vi "AutoFollowRelativeTrajectoryNEW.vi"(8 "error in (no error)":errorcluster, 9 "TimeOut (s)":dbl, 10 "End Orientation":dbl, 11 "Trajectory":T1 {"States"."POSE"."ROTATION"."SIN" format="%13.4f"; "States"."POSE"."ROTATION"."COS" format="%13.4f"; "States"."POSE"."ROTATION"."VALUE" format="%13.4f"; "States"."POSE"."TRANSLATION"."Y" format="%14.3f"; "States"."POSE"."TRANSLATION"."X" format="%14.3f"; "TotalTImeSecs" format="%20.3f"}) -> (0 "error out":errorcluster)   [LabVIEW 2023]
doc: "Wrapper class for drive straight"
uses:
  <vilib>/Rock Robotics/WPI/ThirdParty/JAS_Junk/TrajLib/TypeDef/TRAJECTORY.ctl
  <vilib>/Rock Robotics/WPI/ThirdParty/JAS_Junk/TrajLib/TypeDef/TRAJ_STATE.ctl
  <vilib>/Rock Robotics/WPI/ThirdParty/JAS_Junk/TrajLib/TypeDef/POSE2D.ctl
  <vilib>/Rock Robotics/WPI/ThirdParty/JAS_Junk/TrajLib/TypeDef/TRANSLATION2D.ctl
  <vilib>/Rock Robotics/WPI/ThirdParty/JAS_Junk/TrajLib/TypeDef/ROTATION2D.ctl
  <vilib>/Rock Robotics/WPI/ThirdParty/JAS_Junk/TrajLib/ChassisSpeeds_New.vi
  <vilib>/Rock Robotics/WPI/ThirdParty/JAS_Junk/TrajLib/Conv_Feet_Meters.vi
  <vilib>/Rock Robotics/WPI/ThirdParty/JAS_Junk/TrajLib/Conv_Deg_Radians.vi
  <vilib>/Utility/semaphor.llb/Obtain Semaphore Reference.vi
  <vilib>/Rock Robotics/WPI/ThirdParty/JAS_Junk/TrajLib/Timer_Reset.vi
  Drive/DriveGlobal.vi
  <vilib>/Rock Robotics/WPI/ThirdParty/JAS_Junk/TrajLib/Trajectory_Library.lvlib
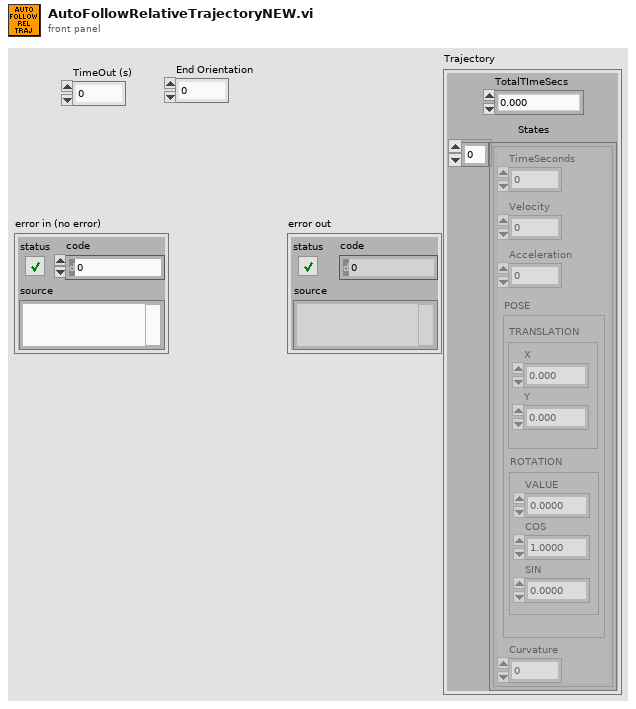
[diagram p1: front panel]
types:
  T1 = typedef "Trajectory_Library.lvlib/TRAJECTORY.ctl" = cluster{"TotalTImeSecs":dbl, "States":T2[]}
  T2 = typedef "Trajectory_Library.lvlib/TRAJ_STATE.ctl" = cluster{"TimeSeconds":dbl, "Velocity":dbl, "Acceleration":dbl, "POSE":T3, "Curvature":dbl}
  T3 = typedef "Trajectory_Library.lvlib/POSE2D.ctl" = cluster{"TRANSLATION":T4, "ROTATION":T5}
  T4 = typedef "Trajectory_Library.lvlib/TRANSLATION2D.ctl" = cluster{"X":dbl, "Y":dbl}
  T5 = typedef "Trajectory_Library.lvlib/ROTATION2D.ctl" = cluster{"VALUE":dbl, "COS":dbl, "SIN":dbl}
  T6 = typedef "Trajectory_Library.lvlib/TIMER.ctl" = cluster{"StartTime":dbl, "Accumulated TIme":dbl, "Running":bool, "semaphore":T7}
  T7 = typedef "Semaphore RefNum" = refnum<k1>
  T8 = typedef "Trajectory_Library.lvlib/CHASSIS_SPEEDS.ctl" = cluster{"vX":dbl, "vY":dbl, "vOmega":dbl}
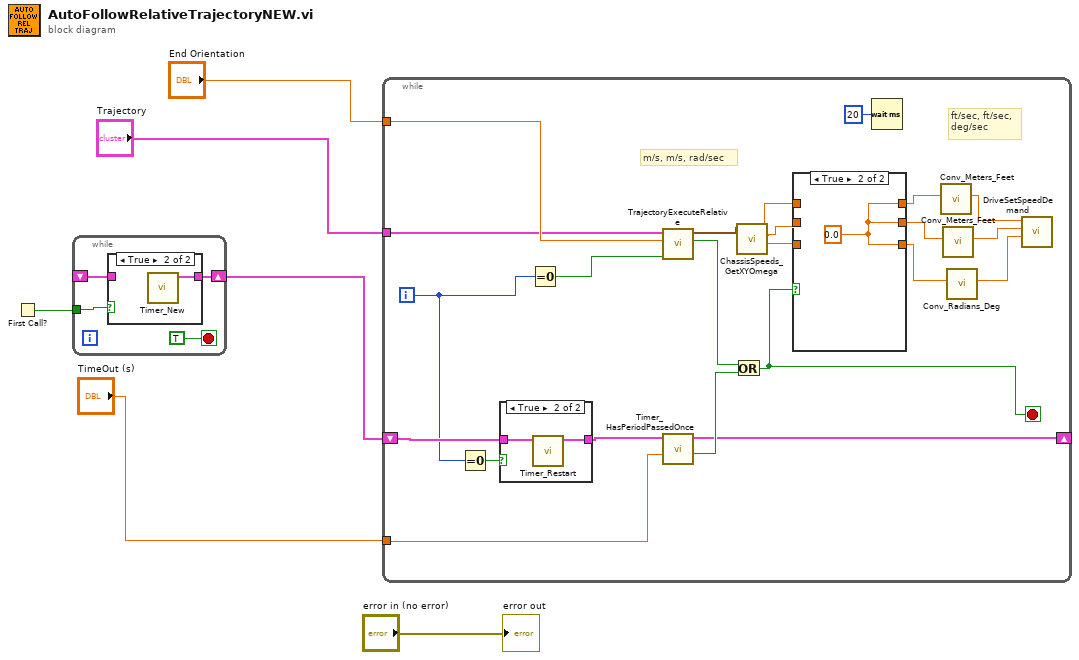
[diagram p0: block diagram]
diagram:
  n1 = First Call?() -> (First Call?: T/F=w2:bool)
  n2 = while {
    tunnel: w2 -> [w7]
    shift-right: [w10] -> w1
    shift-left: _ -> [w8]
    stop <- TRUE stop-if-true
    n3 = case shown="True" w7 {
      tunnel: [w11 w12] -> w10
      tunnel: w8 -> [w11 _]
      frame False {
      }
      frame True {
        n4 = call <vilib>:"Timer_New.vi"() -> ("TIMER"=w12:T6)  [unwired: 11 in]
      }
    }
  }
  n5 = while {
    tunnel: "TimeOut (s)" -> [w35]
    tunnel: "Trajectory" -> [w31]
    tunnel: "End Orientation" -> [w32]
    shift-right: [w15] -> _
    shift-left: w1 -> [w14]
    i -> [w13]
    stop <- w18 stop-if-true
    # "ft/sec, ft/sec,\ndeg/sec"
    # "m/s, m/s, rad/sec"
    n6 = Equal To 0?(x=w13) -> (x = 0?=w17:bool)
    n7 = case shown="True" w17 {
      tunnel: w14 -> [w36 w38]
      tunnel: [w36 w37] -> w16
      frame False {
      }
      frame True {
        n8 = call <vilib>:"Timer_Restart.vi"("in Timer"=w38) -> ("out Timer"=w37:T6)  [unwired: 10 in]
      }
    }
    n9 = Equal To 0?(x=w13) -> (x = 0?=w30:bool)
    n10 = call "TrajectoryExecuteRelative.vi"("Init"=w30, "End Relative\nOrientation Deg"=w32, "Trajectory"=w31) -> ("Done"=w29:bool, "Chassis Velocity Target Met,Met,Rad"=w25:T8)  [unwired: 6 in, 1 out]
    n11 = call <vilib>:"Timer_HasPeriodPassedOnce.vi"("Period"=w35, "in Timer"=w16) -> ("Expired"=w34:bool, "out Timer"=w15:T6)  [unwired: 7 in, 1 out]
    n12 = Or(x=w29, y=w34) -> (x .or. y?=w18:bool)
    n13 = call <vilib>:"ChassisSpeeds_GetXYOmega.vi"("CHASSIS"=w25) -> ("vAngular"=w28:dbl, "vY"=w27:dbl, "vX"=w26:dbl)  [unwired: 8 in]
    n14 = case shown="True" w18 {
      tunnel: w26 -> [w41 _]
      tunnel: w27 -> [w40 _]
      tunnel: w28 -> [w39 _]
      tunnel: [w41 w42] -> w24
      tunnel: [w40 w42] -> w22
      tunnel: [w39 w42] -> w20
      frame False {
      }
      frame True {
        w42 = 0.0 ("XSpeedDemand")
      }
    }
    n15 = Wait (ms)(milliseconds to wait=u32 20) -> ()  [unwired: 1 out]
    n16 = call <vilib>:"Conv_Meters_Feet.vi"("Meters"=w24) -> ("Feet"=w23:dbl)  [unwired: 10 in]
    n17 = call <vilib>:"Conv_Meters_Feet.vi"("Meters"=w22) -> ("Feet"=w21:dbl)  [unwired: 10 in]
    n18 = call <vilib>:"Conv_Radians_Deg.vi"("Radians"=w20) -> ("Degrees"=w19:dbl)  [unwired: 10 in]
    n19 = call "DriveSetSpeedDemand.vi"("ASpeedDemand (d/s)"=w19, "YSpeedDemand (ft/s)"=w21, "XSpeedDemand (ft/s)"=w23) -> ()  [unwired: 9 in]
  }
  "error out" <- "error in (no error)"
